vi "Get_Alarm_Config.vi"(8 "error in (no error)":errorcluster, 11 "Alarm_Data In":T1) -> (0 "error out":errorcluster, 3 "Alarm_Data Out":T1)   [LabVIEW 2019, in "Alarm_Manager.lvlib"]
uses:
  Alarm_Manager.lvlib
  Alarm_Data.ctl
  Message_Handler/typedef/Alarm_Panel.ctl
  Channel_Temperature_Threshold.ctl
  <vilib>/Utility/config.llb/Read Key (U32).vi
  <vilib>/Utility/config.llb/Read Key (I32).vi
  <vilib>/Utility/config.llb/NI_LVConfig.lvlib
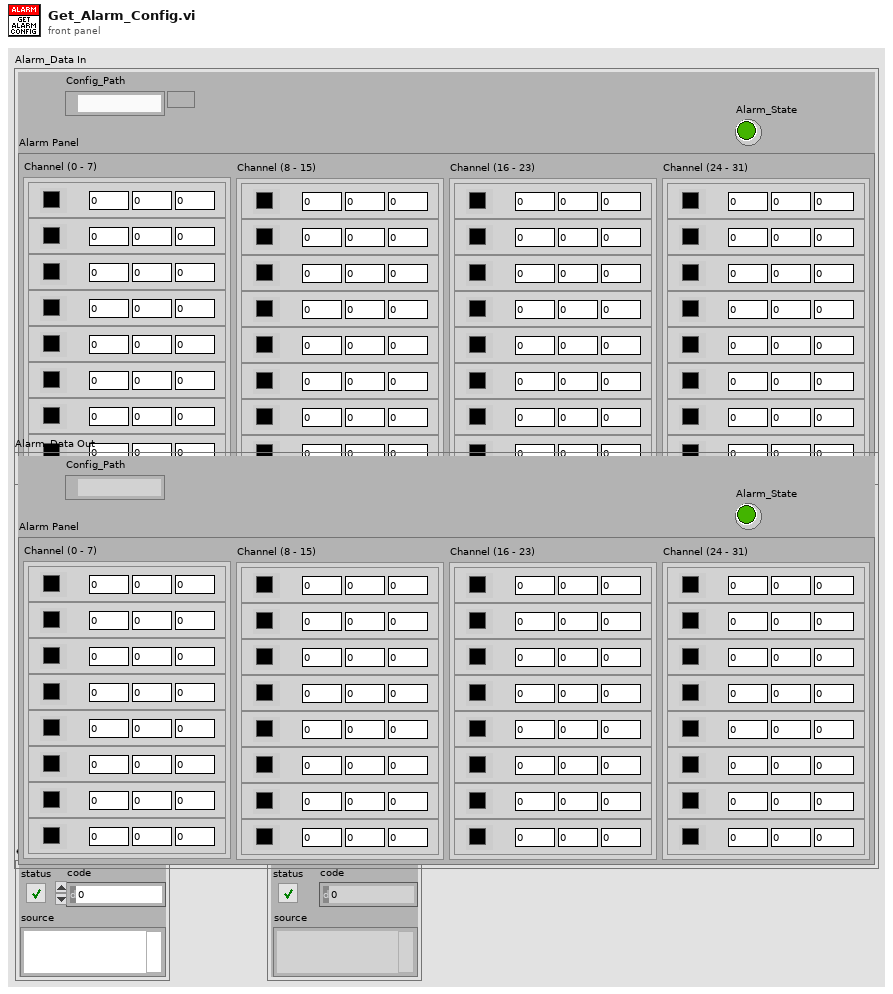
[diagram p1: front panel]
types:
  T1 = typedef "Alarm_Data.ctl" = cluster{"Alarm Panel":T2, "Alarm_State":bool, "Config_Path":path}
  T2 = typedef "Alarm_Panel.ctl" = cluster{"Channel (0 - 7)":cluster{"Channel Temperature Thresholds":T3, "Channel Temperature Thresholds 2":T3, "Channel Temperature Thresholds 3":T3, "Channel Temperature Thresholds 4":T3, "Channel Temperature Thresholds 5":T3, "Channel Temperature Thresholds 6":T3, "Channel Temperature Thresholds 7":T3, "Channel Temperature Thresholds 8":T3}, "Channel (8 - 15)":cluster{"Channel Temperature Thresholds":T3, "Channel Temperature Thresholds 2":T3, "Channel Temperature Thresholds 3":T3, "Channel Temperature Thresholds 4":T3, "Channel Temperature Thresholds 5":T3, "Channel Temperature Thresholds 6":T3, "Channel Temperature Thresholds 7":T3, "Channel Temperature Thresholds 8":T3}, "Channel (16 - 23)":cluster{"Channel Temperature Thresholds":T3, "Channel Temperature Thresholds 2":T3, "Channel Temperature Thresholds 3":T3, "Channel Temperature Thresholds 4":T3, "Channel Temperature Thresholds 5":T3, "Channel Temperature Thresholds 6":T3, "Channel Temperature Thresholds 7":T3, "Channel Temperature Thresholds 8":T3}, "Channel (24 - 31)":cluster{"Channel Temperature Thresholds":T3, "Channel Temperature Thresholds 2":T3, "Channel Temperature Thresholds 3":T3, "Channel Temperature Thresholds 4":T3, "Channel Temperature Thresholds 5":T3, "Channel Temperature Thresholds 6":T3, "Channel Temperature Thresholds 7":T3, "Channel Temperature Thresholds 8":T3}}
  T3 = typedef "Channel_Temperature_Threshold.ctl" = cluster{"Min":i32, "Max":i32, "Alarm":i32, "Status":u32}
  T4 = cluster{"Channel Temperature Thresholds":T3, "Channel Temperature Thresholds 2":T3, "Channel Temperature Thresholds 3":T3, "Channel Temperature Thresholds 4":T3, "Channel Temperature Thresholds 5":T3, "Channel Temperature Thresholds 6":T3, "Channel Temperature Thresholds 7":T3, "Channel Temperature Thresholds 8":T3}
  T5 = typedef "NI_LVConfig.lvlib/Config Data RefNum.ctl" = refnum<k1>
  T6 = cluster{"[0]":T3, "[1]":T3, "[2]":T3, "[3]":T3, "[4]":T3, "[5]":T3, "[6]":T3, "[7]":T3}
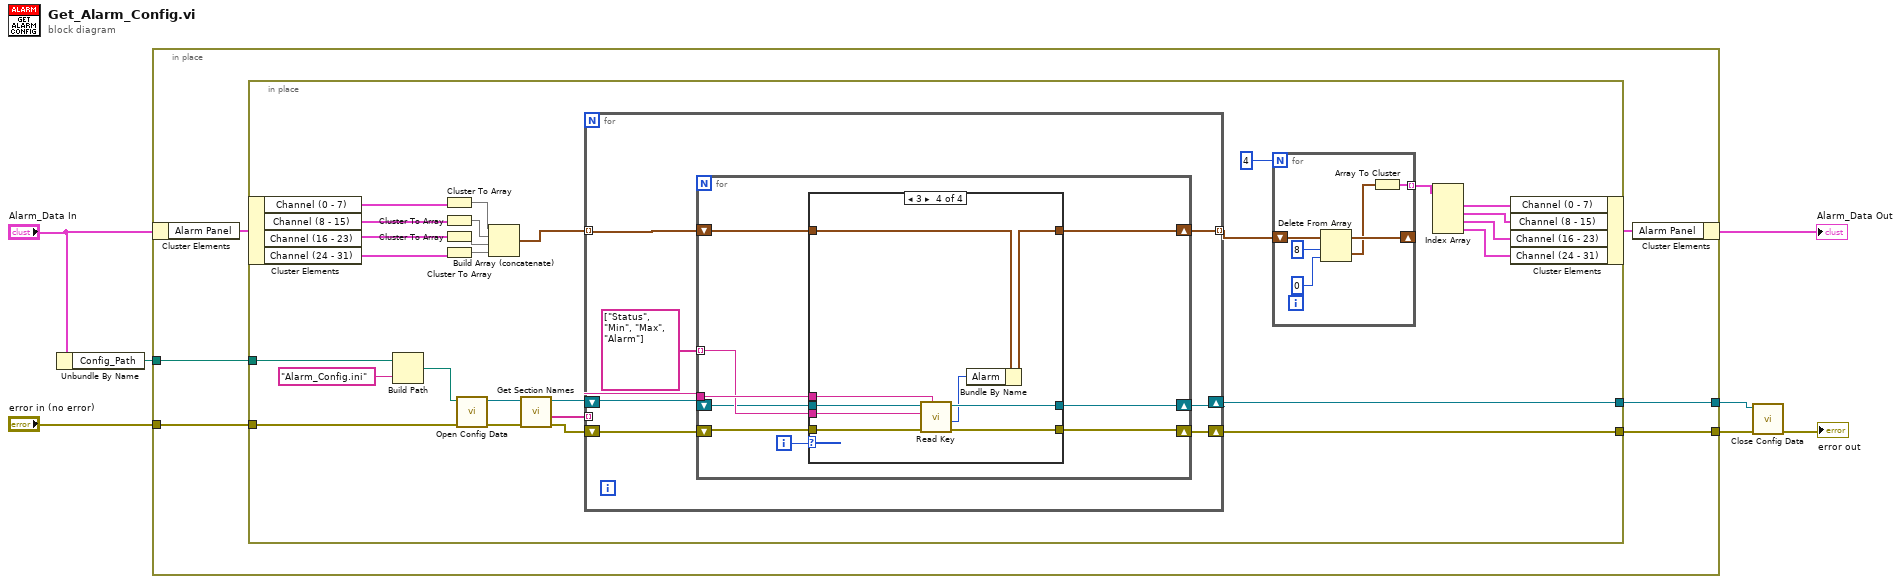
[diagram p0: block diagram]
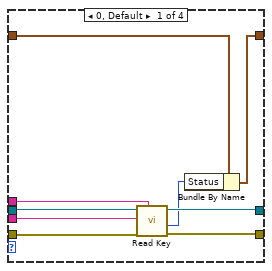
[diagram p2: hidden frame]
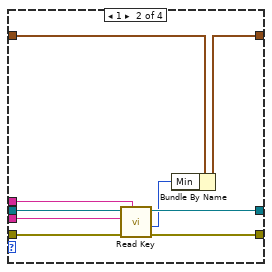
[diagram p3: hidden frame]
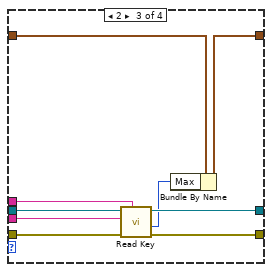
[diagram p4: hidden frame]
diagram:
  n1 = Unbundle By Name("Alarm_Data In") -> ("Config_Path"=w4:path)
  n2 = in-place {
    in-place-border: "error in (no error)" -> [w13]
    in-place-border: w4 -> [w10]
    in-place-border: [w9] -> w3
    in-place-border: [w8] -> w1
    n3 = in-place-cluster #1("Alarm_Data In") -> ("Alarm Panel"=w12:T2)
    n4 = in-place {
      in-place-border: w13 -> [w40]
      in-place-border: w10 -> [w18]
      in-place-border: [w15] -> w9
      in-place-border: [w14] -> w8
      n5 = in-place-cluster #2(w12) -> ("Channel (0 - 7)"=w30:T4, "Channel (8 - 15)"=w29:T4, "Channel (16 - 23)"=w28:T4, "Channel (24 - 31)"=w27:T4)
      n6 = Build Path(base path=w18, name or relative path="Alarm_Config.ini") -> (appended path=w16:path)
      n7 = Cluster To Array(cluster=w30) -> (array=w34:T3[])
      n8 = Cluster To Array(cluster=w29) -> (array=w33:T3[])
      n9 = Cluster To Array(cluster=w28) -> (array=w32:T3[])
      n10 = Cluster To Array(cluster=w27) -> (array=w31:T3[])
      n11 = call <vilib>:"Open Config Data.vi"("error in (no error)"=w40, "configuration file path"=w16) -> ("error out"=w38:errorcluster, "refnum"=w39:T5)  [unwired: 7 in, 1 out]
      n12 = Build Array (concatenate)(w34, w33, w32, w31) -> (w26:T3[])
      n13 = call <vilib>:"Get Section Names.vi"("error in (no error)"=w38, "refnum"=w39) -> ("error out"=w36:errorcluster, "section names"=w37:string[], "refnum out"=w35:T5)  [unwired: 7 in]
      n14 = for {
        tunnel: w37 -> [w54] mode=indexing
        shift-right: [w52] -> w15
        shift-left: w36 -> [w53]
        shift-right: [w50] -> w14
        shift-left: w35 -> [w51]
        tunnel: w26 -> [w48] mode=indexing
        tunnel: [w47] -> w23 mode=indexing
        n15 = for {
          tunnel: w54 -> [w63]
          tunnel: string[] ["Status", "Min", "Max", "Alarm"] -> [w62] mode=indexing
          shift-right: [w60] -> w52
          shift-left: w53 -> [w61]
          shift-right: [w58] -> w50
          shift-left: w51 -> [w59]
          shift-right: [w55] -> w47
          shift-left: w48 -> [w56]
          i -> [w57]
          n16 = case shown="3" w57 {
            tunnel: w63 -> [w68 w81 w90 w99]
            tunnel: w62 -> [w67 w80 w89 w98]
            tunnel: w61 -> [w72 w79 w88 w97]
            tunnel: [w71 w78 w87 w96] -> w60
            tunnel: w59 -> [w69 w77 w86 w95]
            tunnel: [w70 w76 w85 w94] -> w58
            tunnel: w56 -> [w66 w75 w84 w93]
            tunnel: [w64 w73 w82 w91] -> w55
            frame 0, Default {
              n17 = call-poly <vilib>:"Read Key.vi"("section"=w68, "error in (no error)"=w72, "key"=w67, "refnum"=w69) -> ("error out"=w71:errorcluster, "value"=w65:u32, "refnum out"=w70:T5)  [unwired: 4 in, 1 out]
              n18 = Bundle By Name(cluster=w66, "Status"=w65) -> (w64:T3)
            }
            frame 1 {
              n19 = call-poly <vilib>:"Read Key.vi"("section"=w81, "error in (no error)"=w79, "key"=w80, "refnum"=w77) -> ("error out"=w78:errorcluster, "value"=w74:i32, "refnum out"=w76:T5)  [unwired: 4 in, 1 out]
              n20 = Bundle By Name(cluster=w75, "Min"=w74) -> (w73:T3)
            }
            frame 2 {
              n21 = call-poly <vilib>:"Read Key.vi"("section"=w90, "error in (no error)"=w88, "key"=w89, "refnum"=w86) -> ("error out"=w87:errorcluster, "value"=w83:i32, "refnum out"=w85:T5)  [unwired: 4 in, 1 out]
              n22 = Bundle By Name(cluster=w84, "Max"=w83) -> (w82:T3)
            }
            frame 3 {
              n23 = call-poly <vilib>:"Read Key.vi"("section"=w99, "error in (no error)"=w97, "key"=w98, "refnum"=w95) -> ("error out"=w96:errorcluster, "value"=w92:i32, "refnum out"=w94:T5)  [unwired: 4 in, 1 out]
              n24 = Bundle By Name(cluster=w93, "Alarm"=w92) -> (w91:T3)
            }
          }
        }
      }
      n25 = for {
        N: 4 -> [_]
        shift-right: [w44] -> _
        shift-left: w23 -> [w46]
        tunnel: [w41] -> w25 mode=indexing
        n26 = Delete From Array(array=w46, length=8, index=0) -> (deleted portion=w42:T3[], array with subset deleted=w44:T3[])
        n27 = Array To Cluster(array=w42) -> (cluster=w41:T6)
      }
      n28 = Index Array(array=w25) -> (element #1=w19:T6, element #2=w20:T6, element #3=w21:T6, element #4=w22:T6)  [unwired: 4 in]
      n29 = in-place-cluster #2("Channel (0 - 7)"=w19, "Channel (8 - 15)"=w20, "Channel (16 - 23)"=w21, "Channel (24 - 31)"=w22) -> (w11:T2)
    }
    n30 = in-place-cluster #1("Alarm Panel"=w11) -> (→"Alarm_Data Out":T1)
  }
  n31 = call <vilib>:"Close Config Data.vi"("error in (no error)"=w3, "refnum"=w1) -> ("error out"=→"error out":errorcluster)  [unwired: 8 in, 1 out]
